vi "SetBitPos.vi"(1 "Datain":u8, 2 "Mask":u8, 3 "Reg data":u8) -> (0 "Data":u16)   [LabVIEW 2022 SP3, in "BME680.lvlib" / "BME680.lvclass"]
uses:
  BME680.lvclass
  BME680.lvclass/BME680.ctl
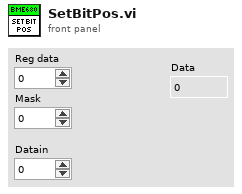
[diagram p1: front panel]
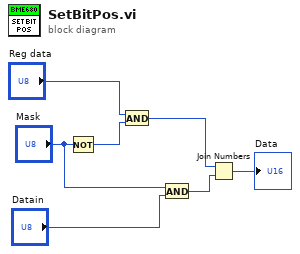
[diagram p0: block diagram]
diagram:
  n1 = Not(x="Mask") -> (.not. x?=w6:u8)
  n2 = And(x="Reg data", y=w6) -> (x .and. y?=w5:u8)
  n3 = And(x="Mask", y="Datain") -> (x .and. y?=w4:u8)
  n4 = Join Numbers(hi=w5, lo=w4) -> ((hi.lo)=→"Data":u16)
